vi "get all paths in variant.vi"(8 "error in (no error)":errorcluster, 11 "Variant":variant) -> (0 "error out":errorcluster, 1 "structure":bool[](array[boolean]), 2 "paths":string[](array[string]))   [LabVIEW 2016, in "JSON Value.lvclass"]
uses:
  JSON Value.lvclass
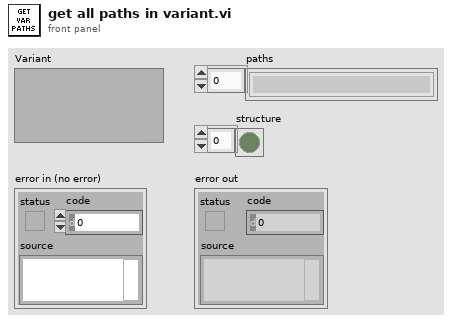
[diagram p1: front panel]
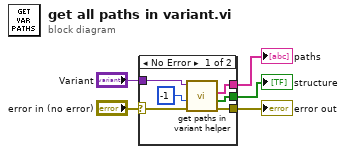
[diagram p0: block diagram]
diagram:
  n1 = case shown="No Error" "error in (no error)" {
    selector: "error in (no error)" -> [w11 w12]
    tunnel: [w10 w12] -> w4
    tunnel: "Variant" -> [w8 _]
    tunnel: [w9 _] -> w2
    tunnel: [w6 _] -> w1
    frame No Error {
      n2 = call "get paths in variant helper.vi"("error in (no error)"=w11, "index"=-1, "variant"=w8) -> ("error out"=w10:errorcluster, "structure"=w6:bool[], "paths"=w9:string[])  [unwired: 6 in]
    }
    frame Error {
    }
  }
  "error out" <- w4
  "paths" <- w2
  "structure" <- w1
